vi "NameWires.vi"(11 "Wires[]":refnum<vi>[](array[refnum])) -> (3 "CodeElements":refnum<class "CodeElement.lvclass">[](array[class]))   [LabVIEW 2017]
uses:
  CodeElements/Base/CodeElement.lvclass
  CodeElements/Variable_Declaration/Variable_Declaration.lvclass
  E:/Code_Generator/CodeElements/Base/CodeElement.lvclass
  CodeElements/Constant_Decl_Def_class/Constant_Decl_Def.lvclass
  CodeElements/SetInputValue_class/SetInputValue.lvclass
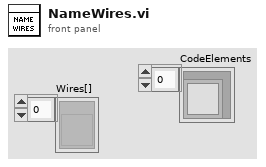
[diagram p1: front panel]
types:
  T1 = typedef "LVPositionTypeDef.ctl" = cluster{"Left":i32, "Top":i32}
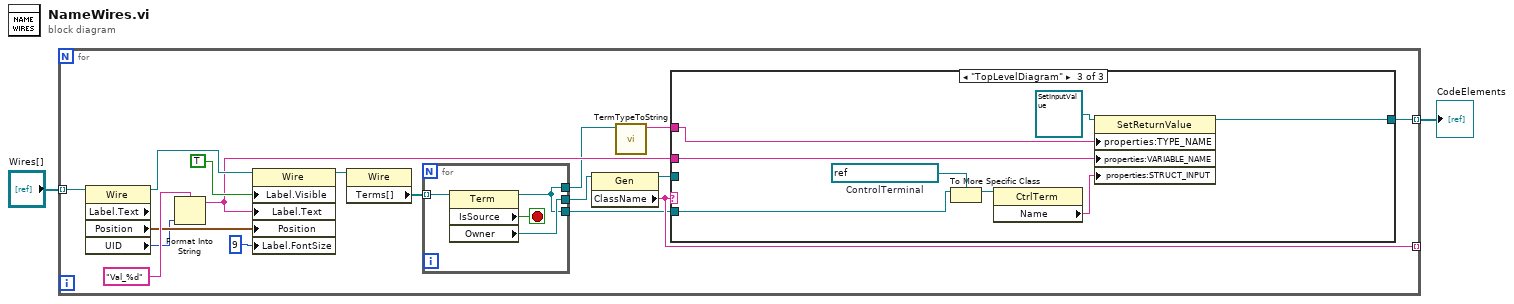
[diagram p0: block diagram]
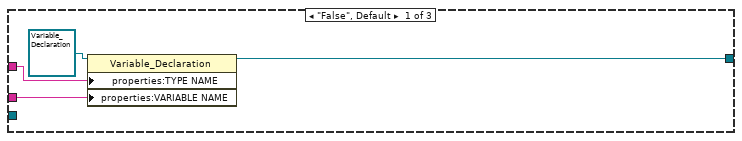
[diagram p2: hidden frame]
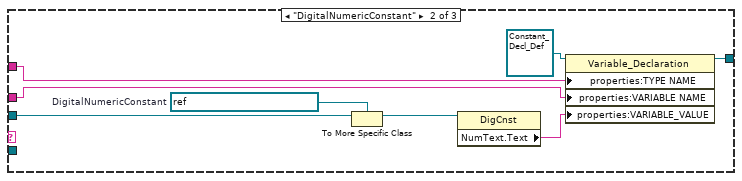
[diagram p3: hidden frame]
diagram:
  n1 = for {
    tunnel: "Wires[]" -> [w19] mode=indexing
    tunnel: [w10] -> w1 mode=indexing
    tunnel: [w5] -> _ mode=indexing
    n2 = property class="Wire" props=["Label", "Text", "Position", "UID"](reference=w19) -> (reference out=w18:refnum<vi>, "Position"=w16:T1, "UID"=w3:i32)  [unwired: 1 in, 2 out]
    n3 = Format Into String(format string="Val_%d", w3) -> (resulting string=w11:string)  [unwired: 2 in, 1 out]
    n4 = property class="Wire"(reference=w18, "Label.Visible"=TRUE, "Label.Text"=w11, "Position"=w16, "Label.FontSize"=u32 9 ("Label.Font:Size")) -> (reference out=w13:refnum<vi>)  [unwired: 1 in, 1 out]
    n5 = property class="Wire"(reference=w13) -> ("Terms[]"=w9:refnum<vi>[])  [unwired: 1 in, 2 out]
    n6 = for {
      tunnel: w9 -> [w43] mode=indexing
      tunnel: [w40] -> w8
      tunnel: [w41] -> w7
      tunnel: [w40] -> w4
      stop <- w42 stop-if-true
      n7 = property class="Term"(reference=w43) -> (reference out=w40:refnum<vi>, "IsSource"=w42:bool, "Owner"=w41:refnum<vi>)  [unwired: 1 in, 1 out]
    }
    n8 = property class="Gen"(reference=w7) -> (reference out=w6:refnum<vi>, "ClassName"=w5:string)  [unwired: 1 in, 1 out]
    n9 = call "TermTypeToString.vi"("Terminal in"=w8) -> ("Name"=w12:string)  [unwired: 10 in]
    n10 = case shown="\"TopLevelDiagram\"" w5 {
      tunnel: w12 -> [w22 w27 w35]
      tunnel: w11 -> [w21 w26 w34]
      tunnel: [w20 w24 w32] -> w10
      tunnel: w6 -> [_ w31 _]
      tunnel: w4 -> [_ _ w37]
      frame "False", Default {
        n11 = property class="Variable_Declaration"(reference=refnum<class "Variable_Declaration.lvclass"> refnum ("Variable_Declaration"), "properties:TYPE NAME"=w22, "properties:VARIABLE NAME"=w21) -> (reference out=w20:refnum<class "Variable_Declaration.lvclass">)  [unwired: 1 in, 1 out]
      }
      frame "DigitalNumericConstant" {
        w30 = refnum<vi> refnum  # DigitalNumericConstant
        n12 = To More Specific Class(target class=w30, reference=w31) -> (specific class reference=w29:refnum<vi>)  [unwired: 1 in, 1 out]
        n13 = property class="DigCnst"(reference=w29) -> ("NumText.Text"=w25:string)  [unwired: 1 in, 2 out]
        n14 = property class="Variable_Declaration"(reference=refnum<class "Constant_Decl_Def.lvclass"> refnum ("Variable_Declaration"), "properties:TYPE NAME"=w27, "properties:VARIABLE NAME"=w26, "properties:VARIABLE_VALUE"=w25) -> (reference out=w24:refnum<class "Constant_Decl_Def.lvclass">)  [unwired: 1 in, 1 out]
      }
      frame "TopLevelDiagram" {
        w39 = refnum<vi> refnum  # ControlTerminal
        n15 = To More Specific Class(target class=w39, reference=w37) -> (specific class reference=w38:refnum<vi>)  [unwired: 1 in, 1 out]
        n16 = property class="CtrlTerm"(reference=w38) -> ("Name"=w33:string)  [unwired: 1 in, 2 out]
        n17 = property class="SetReturnValue"(reference=refnum<class "SetInputValue.lvclass"> refnum ("SetReturnValue"), "properties:TYPE_NAME"=w35, "properties:VARIABLE_NAME"=w34, "properties:STRUCT_INPUT"=w33) -> (reference out=w32:refnum<class "SetInputValue.lvclass">)  [unwired: 1 in, 1 out]
      }
    }
  }
  "CodeElements" <- w1
